vi "Drive Forward to Angle.vi"(5 "PID gains":T5, 6 "yaw":dbl format="%.2f", 7 "yaw setpoint":dbl format="%#_13g", 8 "error in (no error)":errorcluster, 9 "Distance":dbl, 10 "rightDistance":T1={"DevStatus"={"status"=FALSE, "code"=0, "source"=""}, "EncoderIndex"=enum."Invalid", "CounterIndex"=enum."Ctr 1", "DistancePerCount"=2.0, "Decoding Type"=enum."4x"}, 11 "leftDistance":T1={"DevStatus"={"status"=FALSE, "code"=0, "source"=""}, "EncoderIndex"=enum."Invalid", "CounterIndex"=enum."Ctr 1", "DistancePerCount"=2.0, "Decoding Type"=enum."4x"}) -> (0 "error out":errorcluster, 1 "yaw output":dbl format="%.2f", 2 "rightDistance":T1, 3 "leftDistance":T1, 4 "Stop":bool)   [LabVIEW 2017]
uses:
  <vilib>/Rock Robotics/WPI/Encoder/WPI_EncoderDevRef.ctl
  <vilib>/Rock Robotics/SystemInterfaces/Encoder/FPGA_EncoderIdx.ctl
  <vilib>/Rock Robotics/SystemInterfaces/Counter/FPGA_CounterCtrSystemIndex.ctl
  <vilib>/Rock Robotics/WPI/Encoder/WPI_EncoderType.ctl
  <vilib>/addons/control/pid/pid.llb/PID (DBL).vi
  <vilib>/addons/control/pid/NI_PID_pid.lvlib
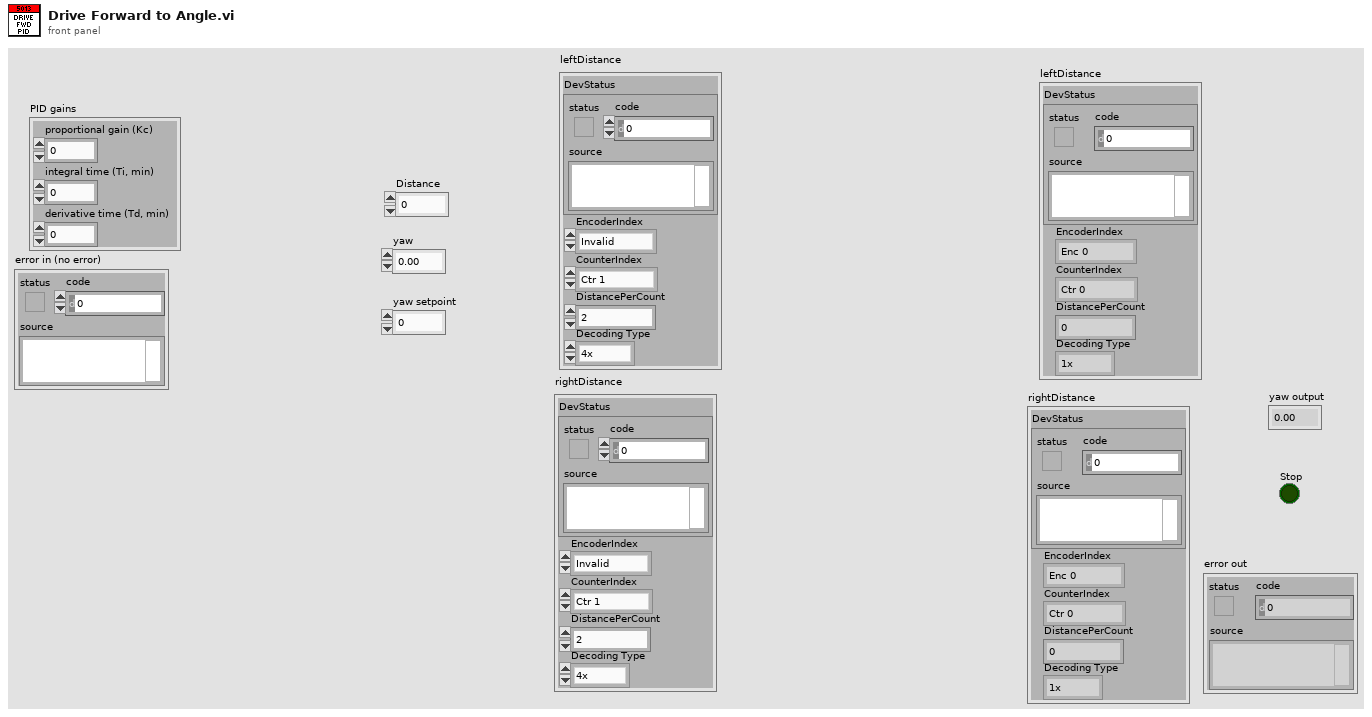
[diagram p1: front panel]
types:
  T1 = typedef "WPI_EncoderDevRef.ctl" = cluster{"DevStatus":errorcluster, "EncoderIndex":T2, "CounterIndex":T3, "DistancePerCount":dbl, "Decoding Type":T4}
  T2 = typedef "FPGA_EncoderIdx.ctl" = enum8{"Enc 0", "Enc 1", "Enc 2", "Enc 3", "Enc 4", "Enc 5", "Enc 6", "Enc 7", "Invalid"}
  T3 = typedef "FPGA_CounterCtrSystemIndex.ctl" = enum8{"Ctr 0", "Ctr 1", "Ctr 2", "Ctr 3", "Ctr 4", "Ctr 5", "Ctr 6", "Ctr 7", "Invalid"}
  T4 = typedef "WPI_EncoderType.ctl" = enum16{"1x", "2x", "4x"}
  T5 = cluster{"proportional gain (Kc)":dbl, "integral time (Ti, min)":dbl, "derivative time (Td, min)":dbl}
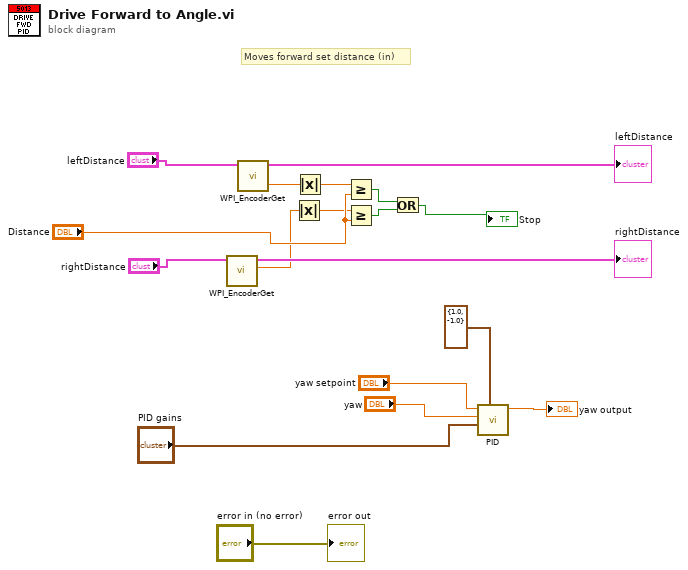
[diagram p0: block diagram]
diagram:
  # "Moves forward set distance (in)"
  n1 = call <vilib>:"WPI_EncoderGet.vi"("EncoderDevRef"="rightDistance") -> ("Distance"=w11:dbl, "EncoderDevRef"=→"rightDistance":T1)  [unwired: 5 in, 4 out]
  n2 = call <vilib>:"WPI_EncoderGet.vi"("EncoderDevRef"="leftDistance") -> ("Distance"=w12:dbl, "EncoderDevRef"=→"leftDistance":T1)  [unwired: 5 in, 4 out]
  n3 = Absolute Value(x=w11) -> (abs(x)=w7:dbl)
  n4 = Absolute Value(x=w12) -> (abs(x)=w8:dbl)
  n5 = Greater Or Equal?(x=w8, y="Distance") -> (x >= y?=w10:bool)
  n6 = Greater Or Equal?(x=w7, y="Distance") -> (x >= y?=w9:bool)
  n7 = Or(x=w10, y=w9) -> (x .or. y?=→"Stop":bool)
  n8 = call-poly <vilib>:"PID.vi"("output range"=cluster{"output high":dbl, "output low":dbl} {"output high"=1.0, "output low"=-1.0}, "PID gains"="PID gains", "process variable"="yaw", "setpoint"="yaw setpoint") -> ("output"=→"yaw output":dbl)  [unwired: 6 in, 1 out]
  "error out" <- "error in (no error)"
